vi "OpenG Array filter - Scalar Template.vi"() -> ()   [LabVIEW 2018]
panel:
  out "filtered item indices":i32[](array[numeric])
  out "filtered array":variant[](array[variant])
  in  "items to filter":variant
  in  "Array Input":variant[](array[variant])
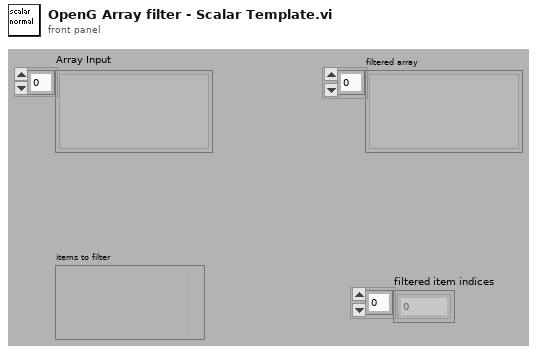
[diagram p1: front panel]
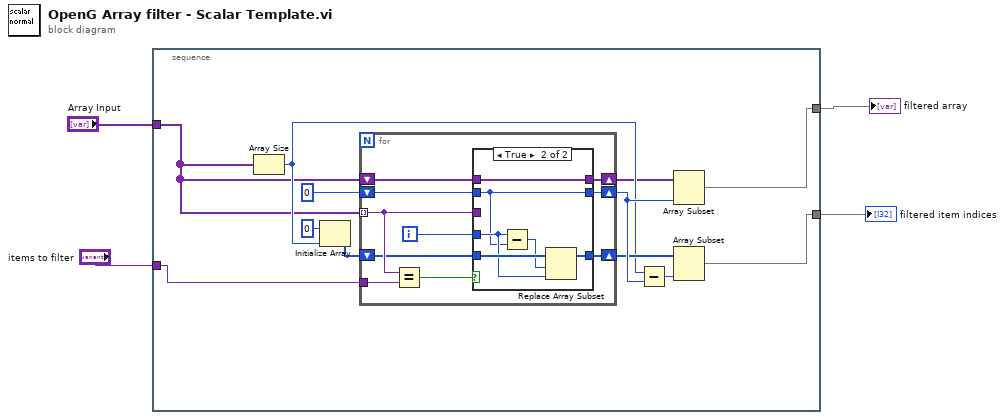
[diagram p0: block diagram]
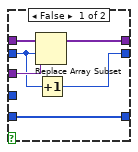
[diagram p2: hidden frame]
diagram:
  n1 = stacked-sequence {
    tunnel: "items to filter" -> [w8]
    tunnel: [w6] -> w3
    tunnel: "Array Input" -> [w7]
    tunnel: [w5] -> w1
    frame #0 {
      n2 = Array Size(array=w7) -> (size(s)=w13:i32)
      n3 = Initialize Array(0 ("Numeric"), w13) -> (w12:i32[])
      n4 = for {
        tunnel: w7 -> [w24] mode=indexing
        shift-right: [w25] -> w10
        shift-left: w7 -> [w26]
        shift-right: [w22] -> w15
        shift-left: 0 -> [w23]
        shift-right: [w20] -> w14
        shift-left: w12 -> [w21]
        tunnel: w8 -> [w19]
        i -> [w18]
        n5 = Equal?(x=w24, y=w19) -> (x = y?=w17:bool)
        n6 = case shown="True" w17 {
          tunnel: w26 -> [w32 w38]
          tunnel: [w31 w38] -> w25
          tunnel: w24 -> [w30 _]
          tunnel: w23 -> [w28 w34]
          tunnel: [w29 w34] -> w22
          tunnel: w21 -> [w27 w37]
          tunnel: [w27 w36] -> w20
          tunnel: w18 -> [_ w35]
          frame False {
            n7 = Replace Array Subset(array=w32, new element=w30, index=w28) -> (w31:variant[])
            n8 = Increment(x=w28) -> (x+1=w29:i32)
          }
          frame True {
            n9 = Subtract(x=w35, y=w34) -> (x-y=w33:i32)
            n10 = Replace Array Subset(array=w37, new element=w35, index=w33) -> (w36:i32[])
          }
        }
      }
      n11 = Subtract(x=w13, y=w15) -> (x-y=w16:i32)
      n12 = Array Subset(array=w10, length=w15) -> (w5:variant[])  [unwired: 1 in]
      n13 = Array Subset(array=w14, length=w16) -> (w6:i32[])  [unwired: 1 in]
    }
  }
  "filtered array" <- w1
  "filtered item indices" <- w3
